vi "Validate Current.vi"(8 "error in (no error)":errorcluster, 10 "Current Setpoint in":dbl, 11 "Acopian in":refnum<class "Acopian.lvclass">) -> (0 "error out":errorcluster, 2 "Current Setpoint out":dbl, 3 "Acopian out":refnum<class "Acopian.lvclass">)   [LabVIEW 2019, in "Acopian.lvlib" / "Acopian.lvclass"]
uses:
  Library/Acopian.lvclass
  C:/Users/rdexter/Documents/Development/Drivers/PPL/PowerSupply.lvlibp/PowerSupply.lvclass
  Library/Acopian.lvclass/Acopian.ctl
  Accessors/Read Max I.vi
  PPL/PowerSupply.lvlibp/Accessors/Read/Read Current Setpoint.vi
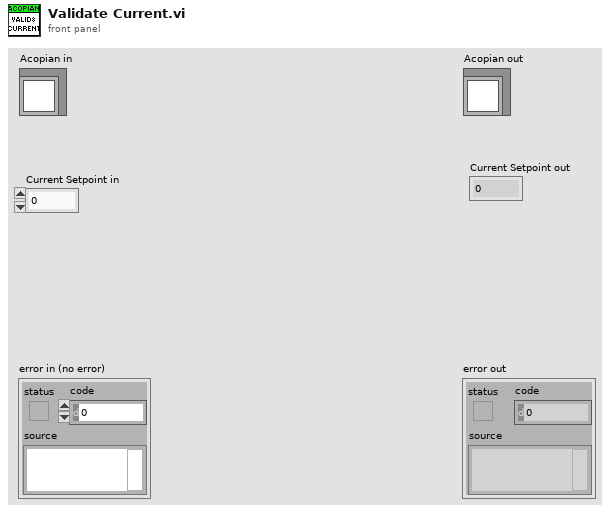
[diagram p1: front panel]
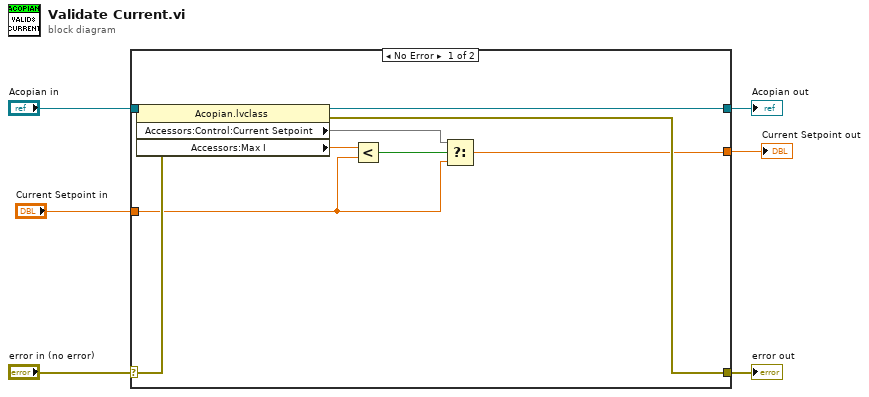
[diagram p0: block diagram]
diagram:
  n1 = case shown="No Error" "error in (no error)" {
    selector: "error in (no error)" -> [w12 w17]
    tunnel: [w9 w17] -> w5
    tunnel: [w10 w16] -> w3
    tunnel: "Acopian in" -> [w15 w16]
    tunnel: [w8 _] -> w2
    tunnel: "Current Setpoint in" -> [w7 _]
    frame No Error {
      n2 = property class="Acopian.lvclass"(reference=w15, error in=w12) -> (reference out=w10:refnum<class "Acopian.lvclass">, error out=w9:errorcluster, "Accessors:Control:Current Setpoint"=w11, "Accessors:Max I"=w14:dbl)
      n3 = Less?(x=w14, y=w7) -> (x < y?=w13:bool)
      n4 = Select(t=w11, s=w13, f=w7) -> (s? t:f=w8:dbl)
    }
    frame Error {
    }
  }
  "error out" <- w5
  "Acopian out" <- w3
  "Current Setpoint out" <- w2
